vi "Initialize.vi"(8 "error in (no error)":errorcluster, 11 "ChromaPowerSupplyModel in":refnum<class "ChromaPowerSupplyModel.lvclass">) -> (0 "error out":errorcluster, 3 "ChromaPowerSupplyModel out":refnum<class "ChromaPowerSupplyModel.lvclass">)   [LabVIEW 2018, in "AcPwrPlugins.lvlib" / "ChromaPowerSupplyModel.lvclass"]
doc: "This VI establishes communication to the instrument and may provide other functions such as reset the instrument or provide a range check."
uses:
  ChromaPowerSupplyModel.lvclass
  Database/DatabaseBaseClass/DatabaseBaseClass.lvclass
  TypeDefs/ChromaPS_ICDAS2Model.ctl
  TypeDefs/ChromaPS_Model2ICDAS.ctl
  ChromaPowerSupplyModel.lvclass/ChromaPowerSupplyModel.ctl
  AcPwrBaseClass/AcPwrBase.lvclass
  <vilib>/addons/database/NI_Database_API.lvlib
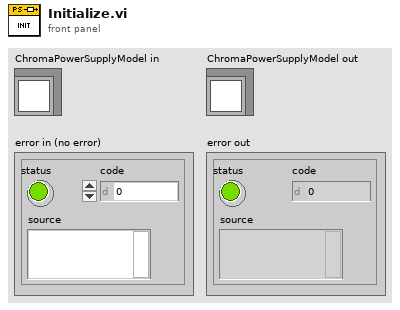
[diagram p1: front panel]
types:
  T1 = typedef "AcPwrPlugins.lvlib/ChromaPowerSupplyModel.lvclass/ChromaPS_Model2ICDAS.ctl" = cluster{"data_id":i32, "voltage":dbl, "current":dbl, "power":dbl, "meas_timestamp":timestamp, "write_timestamp":timestamp, "read_by_icdas":bool, "read_timestamp":timestamp}
  T2 = typedef "AcPwrPlugins.lvlib/ChromaPowerSupplyModel.lvclass/ChromaPS_ICDAS2Model.ctl" = cluster{"data_id":i32, "output_mode":string, "current":dbl, "current_limit_low":dbl, "current_limit_high":dbl, "current_protect":dbl, "current_slew":dbl, "voltage":dbl, "voltage_limit_low":dbl, "voltage_limit_high":dbl, "voltage_protect":dbl, "voltage_slew":dbl, "power_protect":dbl, "write_timestamp":timestamp, "read_by_model":bool, "read_timestamp":timestamp, "meas_interval_ms":u32, "current_slew_rate_infinite":bool}
  T3 = typedef "AcPwrPlugins.lvlib/ChromaPowerSupply.lvclass/Measurements.ctl" = cluster{"Handle":string, "Name":string, "Enabled":bool, "Measurement Value":dbl, "btnMeasFetch":bool, "ProtectionStatusString":string, "Measurement Type":enum16{"Voltage", "Current", "Power"}}[]
  T4 = typedef "AcPwrPlugins.lvlib/ChromaPowerSupply.lvclass/Device(s)Settings.ctl" = cluster{"Phases":cluster{"Handle":string, "Instrument Options":string, "id query (T)":bool, "reset device (T)":bool, "Timing":cluster{"TimingOn":enum16{""}, "Hours":u32, "Minutes":u32, "Seconds":dbl, "CutoffVoltage":dbl}, "Connected":bool, "Output Mode":enum16{"Voltage (DC)", "Current (DC)"}, "Voltage":dbl, "Current":dbl, "High Voltage Limit":dbl, "High Current Limit":dbl, "Power Protect":dbl, "Current Protect":dbl, "Voltage Protect":dbl, "Low Current Limit":dbl, "Low Voltage Limit":dbl, "Current Slew Rate":dbl, "Voltage Slew Rate":dbl, "Current Slew Infinite?":bool}[], "MeasName":string}
  T5 = typedef "AcPwrPlugins.lvlib/ChromaPowerSupplyModel.lvclass/Database Settings.ctl" = cluster{"Data Source":string, "ICDAS to Model Table":string, "Model to ICDAS Table":string}
  T6 = cluster{"Handle":string, "Instrument Options":string, "id query (T)":bool, "reset device (T)":bool, "Timing":cluster{"TimingOn":enum16{""}, "Hours":u32, "Minutes":u32, "Seconds":dbl, "CutoffVoltage":dbl}, "Connected":bool, "Output Mode":enum16{"Voltage (DC)", "Current (DC)"}, "Voltage":dbl, "Current":dbl, "High Voltage Limit":dbl, "High Current Limit":dbl, "Power Protect":dbl, "Current Protect":dbl, "Voltage Protect":dbl, "Low Current Limit":dbl, "Low Voltage Limit":dbl, "Current Slew Rate":dbl, "Voltage Slew Rate":dbl, "Current Slew Infinite?":bool}[]
  T7 = typedef "NI_Database_API.lvlib/Conn ObjectReference.ctl" = refnum<k1>
  T8 = cluster{"Handle":string, "Instrument Options":string, "id query (T)":bool, "reset device (T)":bool, "Timing":cluster{"TimingOn":enum16{""}, "Hours":u32, "Minutes":u32, "Seconds":dbl, "CutoffVoltage":dbl}, "Connected":bool, "Output Mode":enum16{"Voltage (DC)", "Current (DC)"}, "Voltage":dbl, "Current":dbl, "High Voltage Limit":dbl, "High Current Limit":dbl, "Power Protect":dbl, "Current Protect":dbl, "Voltage Protect":dbl, "Low Current Limit":dbl, "Low Voltage Limit":dbl, "Current Slew Rate":dbl, "Voltage Slew Rate":dbl, "Current Slew Infinite?":bool}
  T9 = cluster{"Device Settings":T4, "Database Settings":T5}
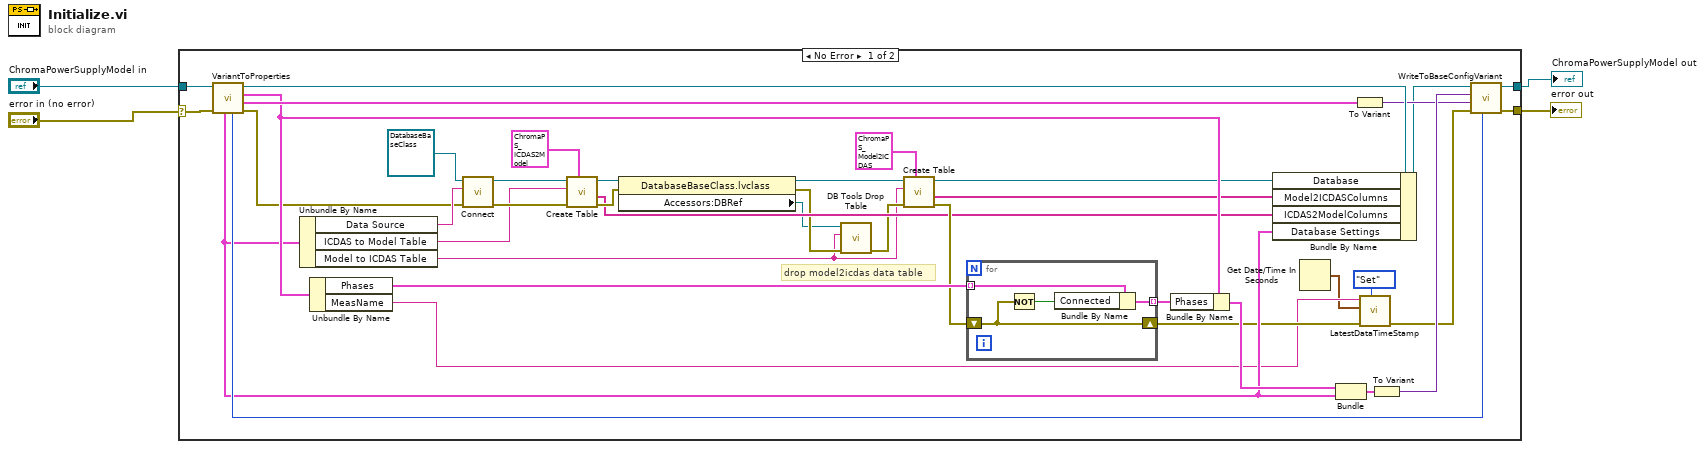
[diagram p0: block diagram]
diagram:
  n1 = case shown="No Error" "error in (no error)" {
    selector: "error in (no error)" -> [w44 w50]
    tunnel: "ChromaPowerSupplyModel in" -> [w36 w49]
    tunnel: [w42 w49] -> w2
    tunnel: [w41 w50] -> w1
    frame No Error {
      # "drop model2icdas data table"
      n2 = call "VariantToProperties.vi"("error in (no error)"=w44, "ChromaPowerSupplyModel in"=w36) -> ("error out"=w30:errorcluster, "Measurements"=w38:T3, "Device Settings"=w33:T4, "ChromaPowerSupplyModel out"=w40:refnum<class "ChromaPowerSupplyModel.lvclass">, "Measurement Refresh Time (ms)"=w37:u32, "Database Settings"=w18:T5)  [unwired: 4 in]
      n3 = Unbundle By Name(w18) -> ("Data Source"=w31:string, "ICDAS to Model Table"=w23:string, "Model to ICDAS Table"=w5:string)
      n4 = Unbundle By Name(w33) -> ("Phases"=w35:T6, "MeasName"=w13:string)
      n5 = call-dynamic "Connect.vi"("error in (no error)"=w30, "Data Source"=w31, "DatabaseBaseClass in"=refnum<class "DatabaseBaseClass.lvclass"> refnum) -> ("error out"=w29:errorcluster, "DatabaseBaseClass out"=w28:refnum<class "DatabaseBaseClass.lvclass">)  [unwired: 7 in]
      n6 = call-dynamic "Create Table.vi"("Cluster In"=T2 {"data_id"=0, "output_mode"="", "current"=0.0, "current_limit_low"=0.0, "current_limit_high"=0.0, "current_protect"=0.0, "current_slew"=0.0, "voltage"=0.0, "voltage_limit_low"=0.0, "voltage_limit_high"=0.0, "voltage_protect"=0.0, "voltage_slew"=0.0, "power_protect"=0.0, "write_timestamp"=timestamp(0 s since 1904-01-01), "read_by_model"=FALSE, "read_timestamp"=timestamp(0 s since 1904-01-01), "meas_interval_ms"=0, "current_slew_rate_infinite"=FALSE} ("ChromaPS_ICDAS2Model"), "error in (no error)"=w29, "Table Name"=w23, "DatabaseBaseClass In"=w28) -> ("error out"=w26:errorcluster, "Column Names"=w16:string[], "DatabaseBaseClass out"=w9:refnum<class "DatabaseBaseClass.lvclass">)  [unwired: 4 in, 1 out]
      n7 = property class="DatabaseBaseClass.lvclass"(reference=w9, error in=w26) -> (reference out=w8:refnum<class "DatabaseBaseClass.lvclass">, error out=w10:errorcluster, "Accessors:DBRef"=w6:T7)
      n8 = call <vilib>:"DB Tools Drop Table.vi"("error in (no error)"=w10, "table"=w5, "connection reference"=w6) -> ("error out"=w7:errorcluster)  [unwired: 5 in, 1 out]
      n9 = call-dynamic "Create Table.vi"("Cluster In"=T1 {"data_id"=0, "voltage"=0.0, "current"=0.0, "power"=0.0, "meas_timestamp"=timestamp(0 s since 1904-01-01), "write_timestamp"=timestamp(0 s since 1904-01-01), "read_by_icdas"=FALSE, "read_timestamp"=timestamp(0 s since 1904-01-01)} ("ChromaPS_Model2ICDAS"), "error in (no error)"=w7, "Table Name"=w5, "DatabaseBaseClass In"=w8) -> ("error out"=w25:errorcluster, "Column Names"=w17:string[], "DatabaseBaseClass out"=w19:refnum<class "DatabaseBaseClass.lvclass">)  [unwired: 4 in, 1 out]
      n10 = for {
        tunnel: w35 -> [w48] mode=indexing
        shift-right: [w46] -> w15
        shift-left: w25 -> [w46]
        tunnel: [w47] -> w34 mode=indexing
        n11 = Not(x=w46) -> (.not. x?=w45:bool)
        n12 = Bundle By Name(cluster=w48, "Connected"=w45) -> (w47:T8)
      }
      n13 = Bundle By Name(cluster=w33, "Phases"=w34) -> (w22:T4)
      n14 = Bundle By Name(cluster=w40, "Database"=w19, "Model2ICDASColumns"=w17, "ICDAS2ModelColumns"=w16, "Database Settings"=w18) -> (w20:refnum<class "ChromaPowerSupplyModel.lvclass">)
      n15 = Get Date/Time In Seconds() -> (seconds since 1Jan1904=w12:timestamp)
      n16 = Bundle("Device Settings"=w22, "Database Settings"=w18) -> (w21:T9)  [unwired: 1 in]
      n17 = To Variant(anything=w38) -> (Variant=w39:variant)
      n18 = call "LatestDataTimeStamp.vi"("Action"=enum16{"Set", "Get"}."Set", "error in (no error)"=w15, "TimeStamp"=w12, "Plugin Name"=w13) -> ("error IO"=w14:errorcluster)  [unwired: 5 in, 2 out]
      n19 = To Variant(anything=w21) -> (Variant=w43:variant)
      n20 = call-dynamic "WriteToBaseConfigVariant.vi"("Measurement Refresh Time (ms)"=w37, "error in (no error)"=w14, "Meas"=w39, "Config"=w43, "ChromaPowerSupplyModel in"=w20) -> ("error out"=w41:errorcluster, "ChromaPowerSupplyModel out"=w42:refnum<class "ChromaPowerSupplyModel.lvclass">)  [unwired: 5 in]
    }
    frame Error {
    }
  }
  "error out" <- w1
  "ChromaPowerSupplyModel out" <- w2
